vi "Convert angle to enum.vi"(10 "Angle":dbl) -> (2 "Miniscan angle":T1)   [LabVIEW 2017]
uses:
  Typedefs/Angle type.ctl
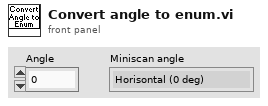
[diagram p1: front panel]
types:
  T1 = typedef "Angle type.ctl" = enum16{"Horisontal (0 deg)", "Vertical (90 deg)", "Any other angle"}
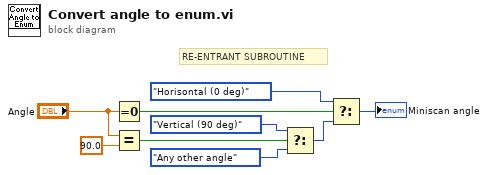
[diagram p0: block diagram]
diagram:
  # "RE-ENTRANT SUBROUTINE"
  n1 = Equal To 0?(x="Angle") -> (x = 0?=w5:bool)
  n2 = Equal?(x="Angle", y=90.0) -> (x = y?=w6:bool)
  n3 = Select(t=Angle_type."Vertical (90 deg)" ("Miniscan angle"), s=w6, f=Angle_type."Any other angle" ("Miniscan angle")) -> (s? t:f=w9:T1)
  n4 = Select(t=Angle_type."Horisontal (0 deg)" ("Miniscan angle"), s=w5, f=w9) -> (s? t:f=→"Miniscan angle":T1)
